vi "ThreeWheelAvg.vi"(7 "Wheel Missing":enum16{"FL", "FR", "RL", "RR"}(ring), 8 "Calculate Rotation?":bool, 9 "Robot Angle (degrees)":dbl(knob) scale=180.0..-180.0, 10 "wheel Y movements (FL, FR, RL, RR)":dbl[](array[numeric]), 11 "wheel X movements (FL, FR, RL, RR)":dbl[](array[numeric])) -> (1 "Rotation":dbl, 2 "Y":dbl, 3 "X":dbl)   [LabVIEW 2014]
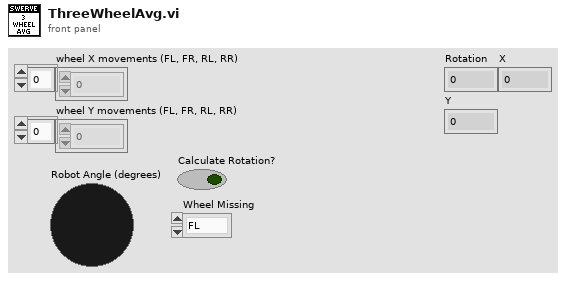
[diagram p1: front panel]
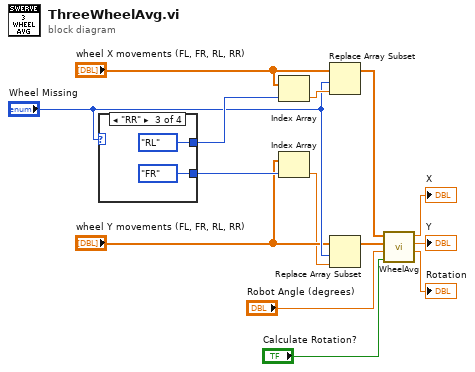
[diagram p0: block diagram]
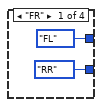
[diagram p2: hidden frame]
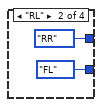
[diagram p3: hidden frame]
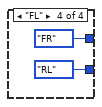
[diagram p4: hidden frame]
diagram:
  n1 = case shown="\"RR\"" "Wheel Missing" {
    tunnel: [enum16{"FL", "FR", "RL", "RR"}."FL" ("Wheel Missing") enum16{"FL", "FR", "RL", "RR"}."RR" ("Wheel Missing") enum16{"FL", "FR", "RL", "RR"}."RL" ("Wheel Missing") enum16{"FL", "FR", "RL", "RR"}."FR" ("Wheel Missing")] -> w7
    tunnel: [enum16{"FL", "FR", "RL", "RR"}."RR" ("Wheel Missing") enum16{"FL", "FR", "RL", "RR"}."FL" ("Wheel Missing") enum16{"FL", "FR", "RL", "RR"}."FR" ("Wheel Missing") enum16{"FL", "FR", "RL", "RR"}."RL" ("Wheel Missing")] -> w6
    frame "FR" {
    }
    frame "RL" {
    }
    frame "RR" {
    }
    frame "FL" {
    }
  }
  n2 = Index Array(array="wheel X movements (FL, FR, RL, RR)", index=w7) -> (element=w8:dbl)
  n3 = Index Array(array="wheel Y movements (FL, FR, RL, RR)", index=w6) -> (element=w1:dbl)
  n4 = Replace Array Subset(array="wheel X movements (FL, FR, RL, RR)", new element=w8, index="Wheel Missing") -> (w5:dbl[])
  n5 = Replace Array Subset(array="wheel Y movements (FL, FR, RL, RR)", new element=w1, index="Wheel Missing") -> (w2:dbl[])
  n6 = call "WheelAvg.vi"("Calculate Rotation?"="Calculate Rotation?", "Robot Angle (degrees)"="Robot Angle (degrees)", "wheel Y movements (FL, FR, RL, RR)"=w2, "wheel X movements (FL, FR, RL, RR)"=w5) -> ("Rotation"=→"Rotation":dbl, "Y"=→"Y":dbl, "X"=→"X":dbl)  [unwired: 5 in]
